vi "Main.vi"(8 "error in (no error)":errorcluster) -> (0 "error out":errorcluster)   [LabVIEW 2020, in "Program.lvclass"]
uses:
  Program.lvclass
  <extravilib>/ChannelInstances/Tag-c(bool,i32,str)/Instantiate.vi
  <extravilib>/ChannelInstances/Tag-c(bool,i32,str)/Endpoint.vi
  <extravilib>/ChannelInstances/Tag-c(bool,i32,str)/EndpointRead.vi
  BubbleTeaShop_class/BubbleTeaShop.lvclass
  Console_class/Console.lvclass
  <extravilib>/ChannelInstances/Tag-c(bool,i32,str).lvlib
panel:
  out "ConsoleText":string
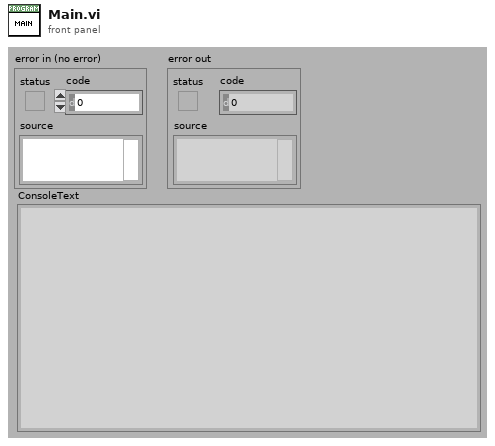
[diagram p1: front panel]
types:
  T1 = typedef "Tag-c(bool,i32,str).lvlib/))Channel.ctl" = refnum<queue>
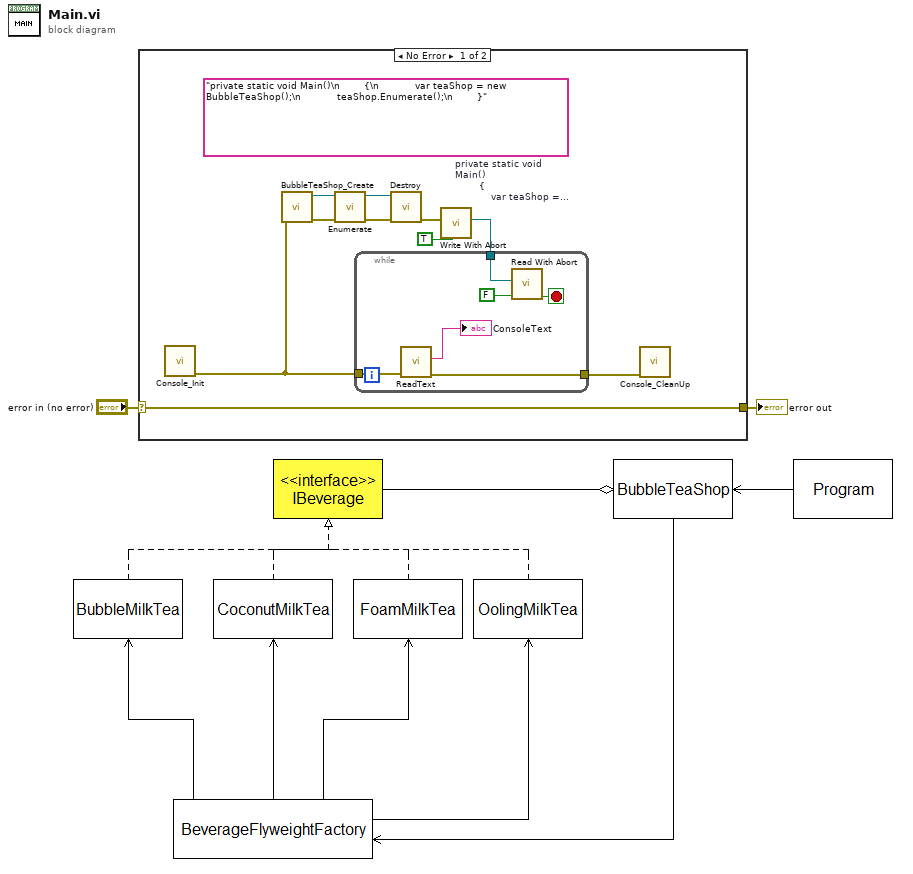
[diagram p0: block diagram]
diagram:
  n1 = case shown="No Error" "error in (no error)" {
    selector: "error in (no error)" -> [w12 w19]
    tunnel: [w12 w19] -> w1
    frame No Error {
      (unwired) "private static void Main()\n        {\n            var teaShop = new BubbleTeaShop();\n            teaShop.Enumerate();\n        }"  # private static void Main()         {             var teaShop = new BubbleTeaShop();             teaShop.Enumerate();         }
      n2 = call "Console_Init.vi"() -> ("Error Out"=w7:errorcluster)  [unwired: 10 in, 1 out]
      n3 = call "BubbleTeaShop_Create.vi"("Error In"=w7) -> ("Error Out"=w11:errorcluster, "reference out"=w10:refnum<class "BubbleTeaShop.lvclass">)  [unwired: 9 in]
      n4 = call-dynamic "Enumerate.vi"("Error In"=w11, "reference in"=w10) -> ("Error Out"=w9:errorcluster, "reference out"=w8:refnum<class "BubbleTeaShop.lvclass">)  [unwired: 7 in, 1 out]
      n5 = call-dynamic "Destroy.vi"("Error In"=w9, "reference in"=w8) -> ("Error Out"=w5:errorcluster)  [unwired: 8 in, 1 out]
      n6 = call <extravilib>:"Write With Abort.vi"("abort"=TRUE, "element"=w5) -> ("channel"=w3:T1)  [unwired: 7 in, 2 out]
      n7 = while {
        tunnel: w7 -> [w18]
        tunnel: [w17] -> w6
        tunnel: w3 -> [w15]
        stop <- w13 stop-if-true
        n8 = call "ReadText.vi"("Error In"=w18) -> ("Error Out"=w17:errorcluster, "TextOut"=→"ConsoleText":string)  [unwired: 9 in]
        n9 = call <extravilib>:"Read With Abort.vi"("abort"=FALSE, "channel"=w15) -> ("aborted?"=w13:bool)  [unwired: 7 in, 2 out]
      }
      n10 = call "Console_CleanUp.vi"("Error In"=w6) -> ()  [unwired: 10 in, 1 out]
    }
    frame Error {
    }
  }
  "error out" <- w1
